vi "Read Results Queue.vi"(8 "error in (no error)":errorcluster, 11 "Launch Measurement and Wait for Result in":refnum<class "Launch Measurement and Wait for Result.lvclass">) -> (0 "error out":errorcluster, 2 "Results Queue":refnum<queue>, 3 "Launch Measurement and Wait for Result out":refnum<class "Launch Measurement and Wait for Result.lvclass">)   [LabVIEW 2017, in "Controller API.lvlib" / "Launch Measurement and Wait for Result.lvclass"]
uses:
  Launch Measurement and Wait for Result.lvclass
  MAL-Framework/user.lib/Common Components/Results/Results.lvclass
  Launch Measurement and Wait for Result.lvclass/Launch Measurement and Wait for Result.ctl
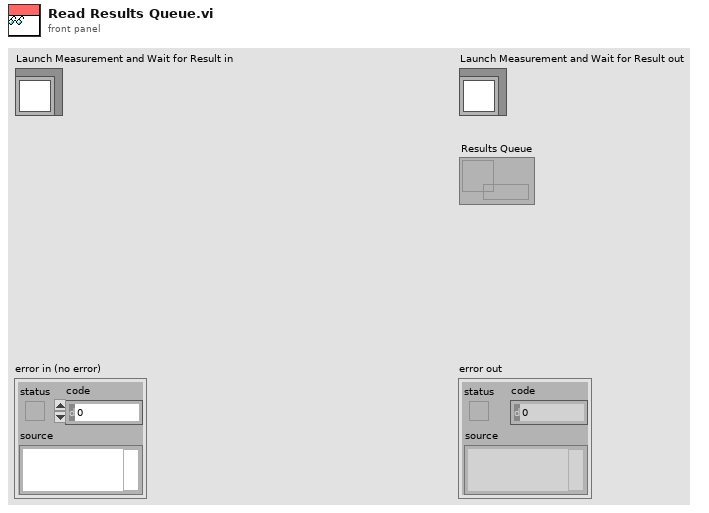
[diagram p1: front panel]
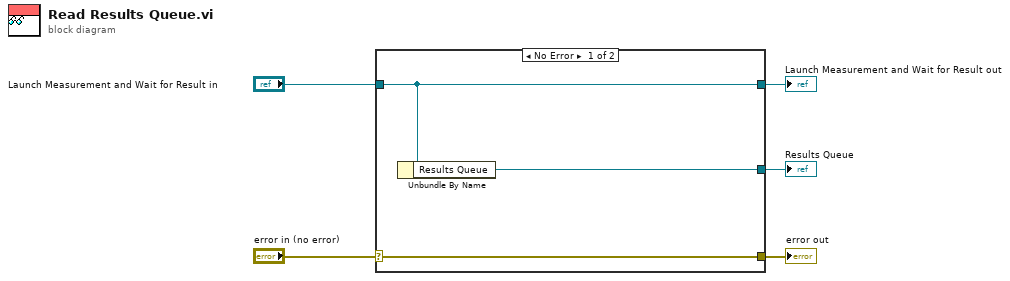
[diagram p0: block diagram]
diagram:
  n1 = case shown="No Error" "error in (no error)" {
    selector: "error in (no error)" -> [w8 w9]
    tunnel: [w8 w9] -> w4
    tunnel: [w7 w10] -> w2
    tunnel: "Launch Measurement and Wait for Result in" -> [w7 w10]
    tunnel: [w6 _] -> w1
    frame No Error {
      n2 = Unbundle By Name(w7) -> ("Results Queue"=w6:refnum<queue>)
    }
    frame Error {
    }
  }
  "error out" <- w4
  "Launch Measurement and Wait for Result out" <- w2
  "Results Queue" <- w1
